vi "Write Numeric.vi"(10 "Numeric":dbl, 11 "Class 1 in":refnum<class "Class 1.lvclass">) -> (3 "Class 1 out":refnum<class "Class 1.lvclass">)   [LabVIEW 2020, in "test_openg_variant.lvlib" / "LVOOP Data.lvlib" / "Class 1.lvclass"]
uses:
  Class 1.lvclass
  Class 1.lvclass/Class 1.ctl
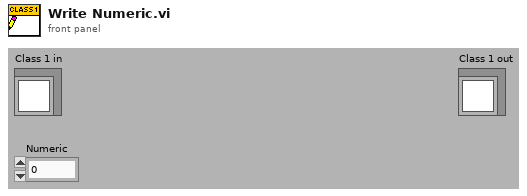
[diagram p1: front panel]
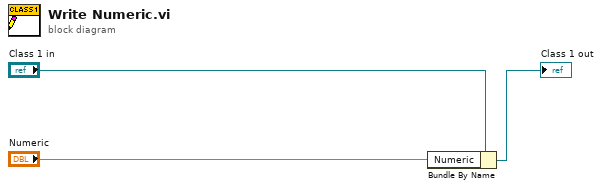
[diagram p0: block diagram]
diagram:
  n1 = Bundle By Name(cluster="Class 1 in", "Numeric"="Numeric") -> (→"Class 1 out":refnum<class "Class 1.lvclass">)
